vi "AppendCode.vi"(6 "New Code":string, 11 "Data In":T1) -> (3 "Data Out":T1)   [LabVIEW 2016]
uses:
  uPythonX/PythonData.ctl
  uPythonX/uPythonX.xctl
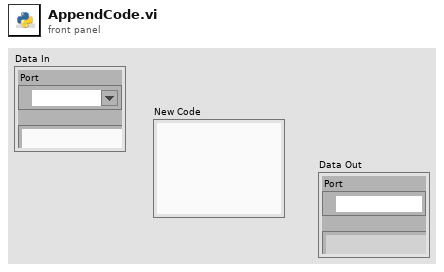
[diagram p1: front panel]
types:
  T1 = typedef "uPythonX.xctl/PythonData.ctl" = cluster{"Port":refnum<visa-resource-name>, "All Code":string}
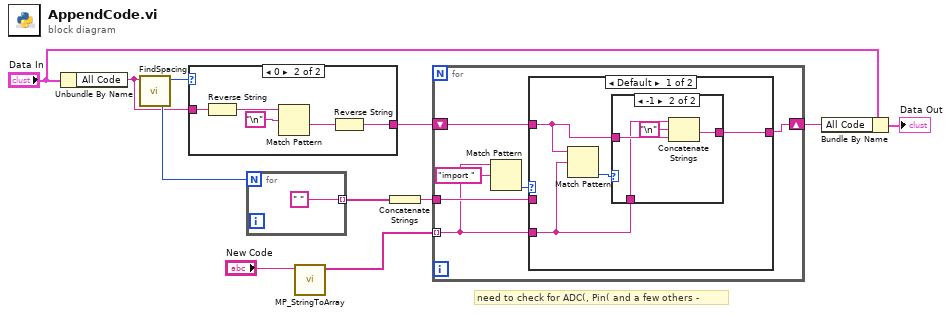
[diagram p0: block diagram]
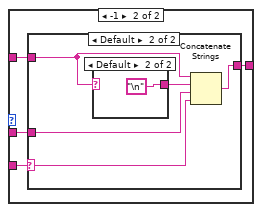
[diagram p4: hidden frame]
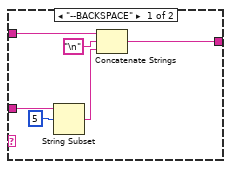
[diagram p5: hidden frame]
diagram:
  # "need to check for ADC(, Pin( and a few others -"
  n1 = Unbundle By Name("Data In") -> ("All Code"=w1:string)
  n2 = call "FindSpacing.vi"("All Code"=w1) -> ("spaces"=w7:i32, "length of cmd"=w3:i32)  [unwired: 8 in, 1 out]
  n3 = case shown="0" w3 {
    tunnel: [w12 w15] -> w2
    tunnel: w1 -> [w12 w17]
    frame Default {
    }
    frame 0 {
      n4 = Reverse String(1:w17) -> (0:w16:string)
      n5 = Match Pattern(string=w16, regular expression="\n") -> (after substring=w13:string)  [unwired: 1 in, 3 out]
      n6 = Reverse String(1:w13) -> (0:w15:string)
    }
  }
  n7 = for {
    N: w7 -> [_]
    tunnel: [" " ("regular expression")] -> w10 mode=indexing
  }
  n8 = call "MP_StringToArray.vi"("write buffer"="New Code") -> ("Array"=w11:string[])  [unwired: 10 in]
  n9 = Concatenate Strings(w10) -> (w5:string)
  n10 = for {
    tunnel: w11 -> [w21] mode=indexing
    tunnel: w5 -> [w23]
    shift-right: [w24] -> w6
    shift-left: w2 -> [w22]
    n11 = Match Pattern(string=w21, regular expression="import ") -> (offset past match=w19:i32)  [unwired: 1 in, 3 out]
    n12 = case shown="Default" w19 {
      tunnel: [w28 w37] -> w24
      tunnel: w23 -> [_ w36]
      tunnel: w22 -> [w27 w35]
      tunnel: w21 -> [w26 w34]
      frame Default {
        n13 = Match Pattern(string=w27, regular expression=w26) -> (offset past match=w25:i32)  [unwired: 1 in, 3 out]
        n14 = case shown="-1" w25 {
          tunnel: [w29 w33] -> w28
          tunnel: w27 -> [w29 w31]
          tunnel: w26 -> [_ w30]
          frame Default {
          }
          frame -1 {
            n15 = Concatenate Strings(w30, "\n" ("string"), w31) -> (w33:string)
          }
        }
      }
      frame -1 {
        n16 = case shown="Default" w34 {
          selector: w34 -> [_ w44]
          tunnel: [w39 w48] -> w37
          tunnel: w36 -> [w43 w47]
          tunnel: w35 -> [w40 w45]
          frame "--BACKSPACE" {
            n17 = String Subset(string=w43, offset (0)=5) -> (substring=w41:string)  [unwired: 1 in]
            n18 = Concatenate Strings(w40, "\n" ("regular expression"), w41) -> (w39:string)
          }
          frame Default {
            n19 = case shown="Default" w45 {
              selector: w45 -> [w49 _]
              tunnel: [w49 "\n" ("string")] -> w46
              frame "" {
              }
              frame Default {
              }
            }
            n20 = Concatenate Strings(w45, w46, w47, w44) -> (w48:string)
          }
        }
      }
    }
  }
  n21 = Bundle By Name(cluster="Data In", "All Code"=w6) -> (→"Data Out":T1)
